vi "6-7.vi"() -> ()   [LabVIEW 2017]
panel:
  out "text":string
  in  "access (0:read/write)":enum16{"read/write", "read-only", "write-only"}(ring)
  in  "operation (0:open)":T1(ring)
  in  "file path (use dialog)":path
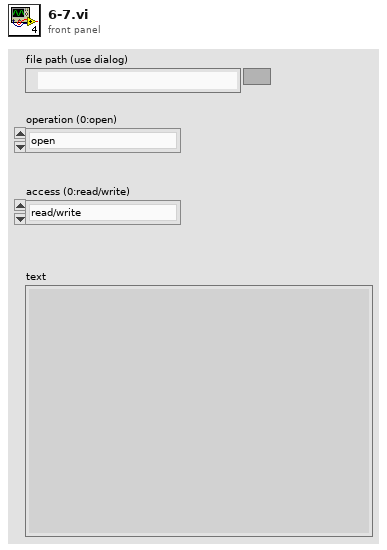
[diagram p1: front panel]
types:
  T1 = enum16{"open", "replace", "create", "open or create", "replace or create", "replace or create with confirmation"}
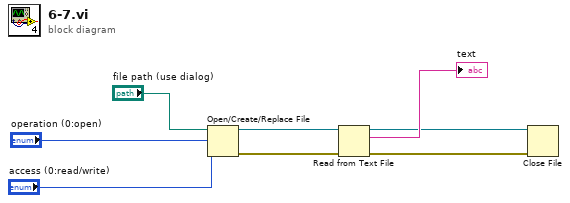
[diagram p0: block diagram]
diagram:
  n1 = Open/Create/Replace File(file path (use dialog)="file path (use dialog)", operation (0:open)="operation (0:open)", access (0:read/write)="access (0:read/write)") -> (refnum out=w5:refnum<file>, error out=w4:errorcluster)  [unwired: 3 in, 1 out]
  n2 = Read from Text File(file (use dialog)=w5, error in=w4) -> (refnum out=w2:refnum<file>, text=→"text":string, error out=w1:errorcluster)  [unwired: 2 in, 1 out]
  n3 = Close File(refnum=w2, error in=w1) -> ()  [unwired: 2 out]
